vi "Memory Benchmark.vi"(5 "Show Cache Lines (F)":bool, 7 "Show Peak Bandwidth (F)":bool, 9 "Transfers (500)":i32=500, 10 "End Size":u64=100000000 format="%.0pB", 11 "Start Size":u64=1000 format="%.0pB") -> (3 "Memory Bandwidth":cluster{"X":dbl[], "Y":dbl[]}[](graph) caption="Memory Bandwidth Plot")   [LabVIEW 2017]
uses:
  UI Pointers.ctl
  Classes/Pointer/Stop/Stop Pointer.lvclass
  Classes/Pointer/Pointer.lvclass
  Classes/Pointer/Read I32.vi
  Classes/Pointer/Write I32.vi
panel:
  out "Progress Message":string
  out "Progress":dbl(slide) scale=0.0..1.0
  out "Peak Throughput":dbl format="%.3pB/s"
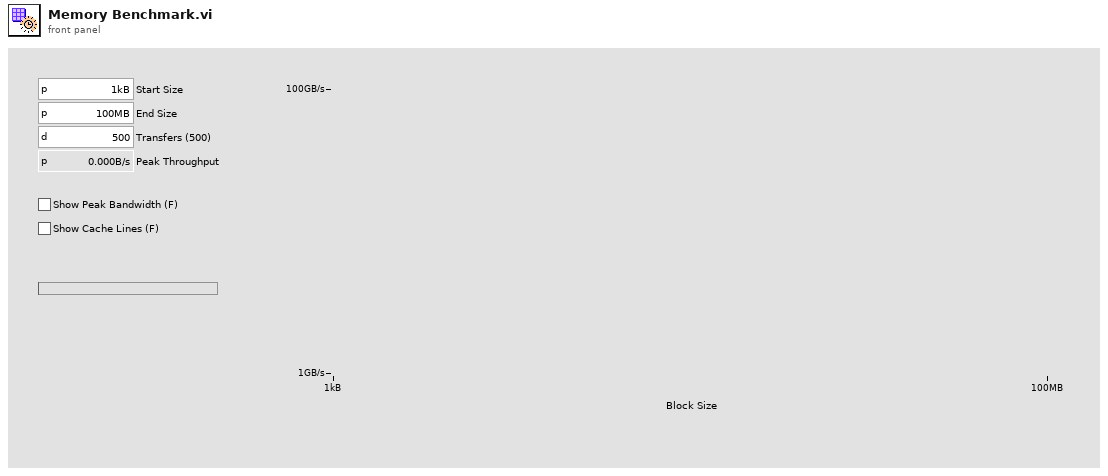
[diagram p1: front panel]
types:
  T1 = typedef "UI Pointers.ctl" = cluster{"Stop Pointer":refnum<class "Stop Pointer.lvclass">, "Iteration Pointer":refnum<class "Pointer.lvclass">}
  T2 = typedef "LVAnnotationListTypeDef.ctl" = cluster{"Name":string, "Color":u32, "Style":u8, "Point Style":u8, "Name Visible":bool, "Allow Drag":bool, "Annotation Mode":u32, "Plot":i32, "Index":i32, "Position":cluster{"X":dbl, "Y":dbl}, "X Scale":u32, "Y Scale":u32, "Show Arrow":bool, "Lock Name":bool, "Plot Area":i32, "Label Offset":cluster{"X":dbl, "Y":dbl}}[]
  T3 = cluster{"Name":string, "Color":u32, "Style":u8, "Point Style":u8, "Name Visible":bool, "Allow Drag":bool, "Annotation Mode":u32, "Plot":i32, "Index":i32, "Position":cluster{"X":dbl, "Y":dbl}, "X Scale":u32, "Y Scale":u32, "Show Arrow":bool, "Lock Name":bool, "Plot Area":i32, "Label Offset":cluster{"X":dbl, "Y":dbl}}
  T4 = cluster{"Name":string, "Color":u32, "Style":u8, "Point Style":u8, "Name Visible":bool, "Allow Drag":bool, "Annotation Mode":u32, "Plot":i32, "Index":i32, "Position":cluster{"X":dbl, "Y":dbl}, "X Scale":u32, "Y Scale":u32, "Show Arrow":bool, "Lock Name":bool, "Plot Area":i32, "Label Offset":cluster{"X":dbl, "Y":dbl}}[]
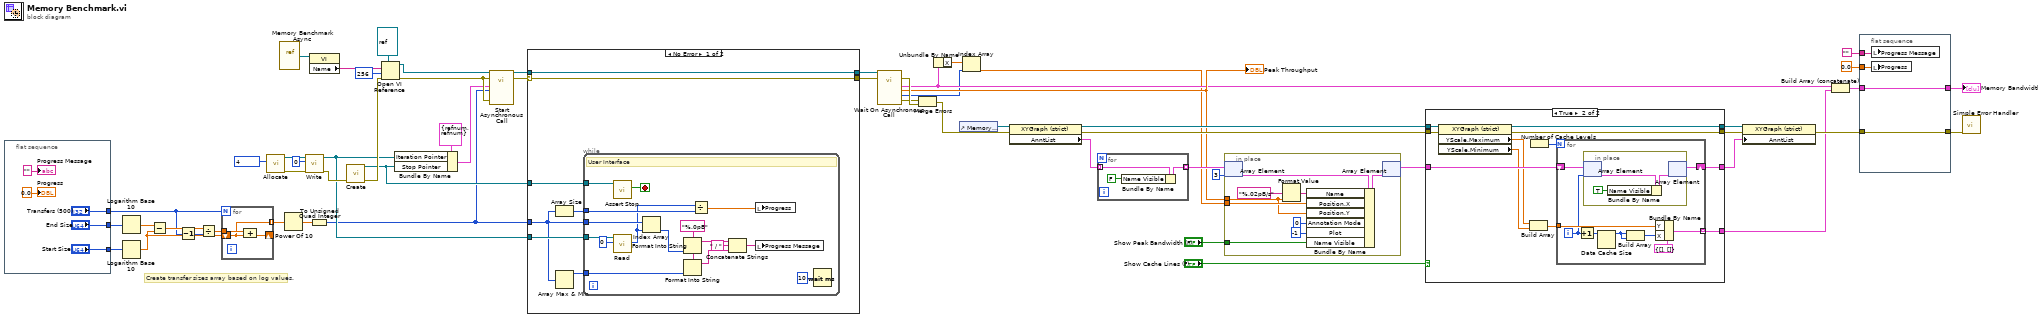
[diagram p0: block diagram]
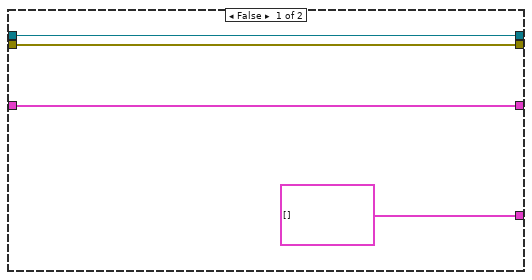
[diagram p3: hidden frame]
diagram:
  # "Create transfer sizes array based on log values."
  n1 = flat-sequence {
    tunnel: ["Start Size"] -> w57
    tunnel: ["End Size"] -> w56
    tunnel: ["Transfers (500)"] -> w51
    frame #0 {
      "Progress" <- 0.0 ("Progress")
      "Progress Message" <- "" ("String")
    }
  }
  n2 = Logarithm Base 10(1:w56) -> (0:w55:dbl)
  n3 = Logarithm Base 10(1:w57) -> (0:w52:dbl)
  n4 = Subtract(x=w55, y=w52) -> (x-y=w54:dbl)
  n5 = Decrement(x=w51) -> (x-1=w50:i32)
  n6 = Divide(x=w54, y=w50) -> (x/y=w53:dbl)
  n7 = for {
    N: w51 -> [_]
    tunnel: w53 -> [w66]
    shift-right: [w65] -> _
    shift-left: w52 -> [w64]
    tunnel: [w64] -> w49 mode=indexing
    n8 = Compound Arithmetic op=ADD(w66, w64) -> (w65:dbl)
  }
  n9 = call "Allocate.vi"("size"=u64 4) -> ("error out"=w34:errorcluster, "Pointer out"=w32:refnum<class "Pointer.lvclass">)  [unwired: 9 in]
  n10 = vi-ref "Memory Benchmark Async.vi"() -> (w24:refnum<vi>)
  n11 = Power Of 10(x=w49) -> (10^x=w48:dbl[])
  n12 = call-poly "Write.vi"("error in (no error)"=w34, "value"=0, "Pointer in"=w32) -> ("error out"=w31:errorcluster, "Pointer out"=w15:refnum<class "Pointer.lvclass">)  [unwired: 5 in, 2 out]
  n13 = property class="VI"(reference=w24) -> ("Name"=w23:string)  [unwired: 1 in, 2 out]
  n14 = To Unsigned Quad Integer(1:w48) -> (0:w5:u64[])
  n15 = call "Create.vi"("error in (no error)"=w31) -> ("error out"=w17:errorcluster, "Stop Pointer"=w16:refnum<class "Stop Pointer.lvclass">)  [unwired: 9 in]
  n16 = Open VI Reference(type specifier VI Refnum (for type only)=refnum<vi> refnum, vi path=w23, options=256, error in (no error)=w17) -> (vi reference=w22:refnum<vi>, error out=w14:errorcluster)  [unwired: 2 in]
  n17 = Bundle By Name(cluster=T1 {"Stop Pointer"=refnum, "Iteration Pointer"=refnum} ("UI Pointers"), "Iteration Pointer"=w15, "Stop Pointer"=w16) -> (w13:T1)
  n18 = call-by-ref "Start Asynchronous Call"(reference=w22, error in=w14, 8:"error in (no error)"=w14, "copy sizes"=w5, "UI Pointers"=w13) -> (reference out=w8:refnum<vi>, error out=w12:errorcluster)  [unwired: 5 in, 4 out]
  n19 = case shown="No Error" w12 {
    selector: w12 -> [w70 w90]
    tunnel: w16 -> [w72 _]
    tunnel: w15 -> [w71 _]
    tunnel: w5 -> [w67 _]
    tunnel: [w70 w90] -> w11
    tunnel: w8 -> [w69 w91]
    tunnel: [w69 w91] -> w7
    frame No Error {
      n20 = Array Size(array=w67) -> (size(s)=w73:i32)
      n21 = Array Max & Min(array=w67) -> (max value=w68:u64)  [unwired: 3 out]
      n22 = while {
        tunnel: w72 -> [w89]
        tunnel: w71 -> [w86]
        tunnel: w67 -> [w84]
        tunnel: w68 -> [w81]
        tunnel: w73 -> [w75]
        stop <- w88 stop-if-true
        w82 = "%.0pB" ("format string")
        # "User Interface"
        n23 = call "Assert Stop.vi"("Stop Pointer in"=w89) -> ("stop?"=w88:bool)  [unwired: 8 in, 2 out]
        n24 = call-poly "Read.vi"("value in"=0, "Pointer in"=w86) -> ("value out"=w74:i32)  [unwired: 6 in, 3 out]
        n25 = Index Array(array=w84, index=w74) -> (element=w80:u64)
        n26 = Format Into String(format string=w82, w80) -> (resulting string=w79:string)  [unwired: 2 in, 1 out]
        n27 = Format Into String(format string=w82, w81) -> (resulting string=w78:string)  [unwired: 2 in, 1 out]
        n28 = Divide(x=w74, y=w75) -> (x/y=w83:dbl)
        n29 = Concatenate Strings(w79, " / " ("string"), w78) -> (w76:string)
        n30 = local write "Progress"(w83) -> ()
        n31 = local write "Progress Message"(w76) -> ()
        n32 = Wait (ms)(milliseconds to wait=u32 10) -> ()  [unwired: 1 out]
      }
    }
    frame Error {
    }
  }
  n33 = call-by-ref "Wait On Asynchronous Call"(reference=w7, error in=w11) -> (error out=w58:errorcluster, 0:"error out"=w10:errorcluster, "peak index"=w4:i32, "peak throughput"=w21:dbl, "results"=w19:cluster{"X":dbl[], "Y":dbl[]})  [unwired: 8 in, 1 out]
  "Peak Throughput" <- w21
  n34 = Merge Errors(w10, w58) -> (w9:errorcluster)
  n35 = Unbundle By Name(w19) -> ("X"=w20:dbl[])
  n36 = control-ref of="Memory Bandwidth"() -> (w44:refnum<vi>)
  n37 = Index Array(array=w20, index=w4) -> (element=w3:dbl)
  n38 = property class="XYGraph (strict)"(reference=w44, error in=w9) -> (reference out=w39:refnum<vi>, error out=w40:errorcluster, "AnntList"=w43:T2)
  n39 = for {
    tunnel: w43 -> [w93] mode=indexing
    tunnel: [w92] -> w41 mode=indexing
    n40 = Bundle By Name(cluster=w93, "Name Visible"=FALSE) -> (w92:T3)
  }
  n41 = in-place {
    in-place-border: w21 -> [w95]
    in-place-border: w3 -> [w99]
    in-place-border: "Show Peak Bandwidth (F)" -> [w96]
    n42 = in-place-array #1(w41, 3) -> (w103:T3)
    n43 = Format Value(format string="%.02pB/s", value (0)=w95) -> (output string=w101:string)  [unwired: 1 in]
    n44 = Bundle By Name(cluster=w103, "Name"=w101, "Position.X"=w99, "Position.Y"=w95, "Annotation Mode"=u32 0, "Plot"=-1, "Name Visible"=w96) -> (w100:T3)
    n45 = in-place-array #1(w100) -> (w45:T4)  [unwired: 1 out]
  }
  n46 = case shown="True" "Show Cache Lines (F)" {
    tunnel: [cluster{"X":dbl[], "Y":dbl[]}[] [] w116] -> w27
    tunnel: w39 -> [w104 w115]
    tunnel: w45 -> [w105 w114]
    tunnel: w40 -> [w106 w113]
    tunnel: [w106 w110] -> w38
    tunnel: [w104 w109] -> w37
    tunnel: [w105 w108] -> w36
    frame False {
    }
    frame True {
      n47 = property class="XYGraph (strict)"(reference=w115, error in=w113) -> (reference out=w109:refnum<vi>, error out=w110:errorcluster, "YScale.Maximum"=w112:dbl, "YScale.Minimum"=w111:dbl)
      n48 = Build Array(w112, w111) -> (w117:dbl[])
      n49 = Number of Cache Levels() -> (w118:i32)
      n50 = for {
        N: w118 -> [_]
        tunnel: w117 -> [w123]
        tunnel: [w122] -> w116 mode=indexing
        shift-right: [w120] -> w108
        shift-left: w114 -> [w121]
        i -> [w119]
        n51 = Increment(x=w119) -> (x+1=w127:i32)
        n52 = in-place {
          n53 = in-place-array #2(w121, w119) -> (w130:T3)
          n54 = Bundle By Name(cluster=w130, "Name Visible"=TRUE) -> (w129:T3)
          n55 = in-place-array #2(w129) -> (w120:T4)  [unwired: 1 out]
        }
        n56 = Data Cache Size(0:w127) -> (4:w125:i32)  [unwired: 1 out]
        n57 = Build Array(w125, w125) -> (w124:i32[])
        n58 = Bundle By Name(cluster=cluster{"X":dbl[], "Y":dbl[]} {"X"=[], "Y"=[]}, "Y"=w123, "X"=w124) -> (w122:cluster{"X":dbl[], "Y":dbl[]})
      }
    }
  }
  n59 = property class="XYGraph (strict)"(reference=w37, error in=w38, "AnntList"=w36) -> (error out=w28:errorcluster)  [unwired: 1 out]
  n60 = Build Array (concatenate)(w19, w27) -> (w30:cluster{"X":dbl[], "Y":dbl[]}[])
  n61 = flat-sequence {
    tunnel: w30 -> [w134]
    tunnel: [w134] -> w29
    tunnel: w28 -> [w133]
    tunnel: [w133] -> w26
    tunnel: "" ("String") -> [w132]
    tunnel: 0.0 ("Progress") -> [w131]
    frame #0 {
      n62 = local write "Progress Message"(w132) -> ()
      n63 = local write "Progress"(w131) -> ()
    }
  }
  n64 = call <vilib>:"Simple Error Handler.vi"("error in (no error)"=w26) -> ()  [unwired: 4 in, 5 out]
  "Memory Bandwidth" <- w29
